vi "Delay.vi"(8 "error in (no error)":errorcluster, 10 "Delay Time (10 ms)":i32=10, 11 "VISA resource name":refnum<visa-resource-name>) -> (0 "error out":errorcluster, 3 "VISA resource name out":refnum<visa-resource-name>)   [LabVIEW 2015, in "IT8900A-E.lvlib"]
uses:
  <instrlib>/IT8900/IT8900A-E.lvlib
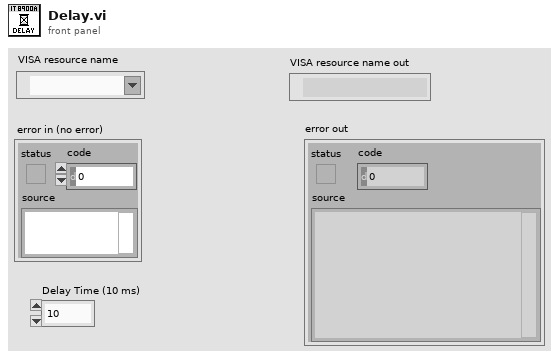
[diagram p1: front panel]
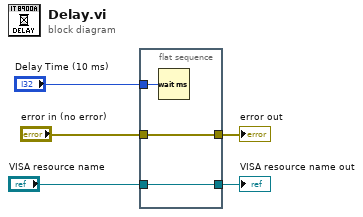
[diagram p0: block diagram]
diagram:
  n1 = flat-sequence {
    tunnel: [w8] -> w4
    tunnel: "VISA resource name" -> [w8]
    tunnel: [w7] -> w3
    tunnel: "error in (no error)" -> [w7]
    tunnel: "Delay Time (10 ms)" -> [w6]
    frame #0 {
      n2 = Wait (ms)(milliseconds to wait=w6) -> ()  [unwired: 1 out]
    }
  }
  "error out" <- w3
  "VISA resource name out" <- w4
